vi "Teleop.vi"(10 "Match Info":T3={"Autonomous Elapsed Seconds"=0.0, "TeleOp Elapsed Seconds"=0.0, "Disabled Elapsed Seconds"=0.0, "Visited Autonomous"=FALSE, "Visited TeleOp"=FALSE, "Visited Disabled"=FALSE, "Autonomous Settings"={"Autonomous Style"=enum."Independent", "VI Refnum"=refnum}}, 11 "Call Context":T4) -> ()   [LabVIEW 2016]
doc: "This VI is called for each TeleOp packet received from the DS where the robot is not disabled. It is often used to read from the joysticks and update I/O or to update setpoints for timed control loops. It should complete and return within 20 milliseconds or it may miss DS packets."
uses:
  <vilib>/Rock Robotics/WPI/DriverStation/WPI_DriverStationDerivedRobotMode.ctl
  <vilib>/Rock Robotics/WPI/DriverStation/WPI_DriverStationMatch Info.ctl
  <vilib>/Rock Robotics/WPI/ThirdParty/Sensors/navX/_TypeDefs/FRIC_navX_DeviceNumbersTypeDef.ctl
  <vilib>/Rock Robotics/WPI/Solenoid/WPI_SolenoidValue.ctl
  <vilib>/Rock Robotics/WPI/Relay/WPI_RelayValue.ctl
  <vilib>/Rock Robotics/WPI/Utilities/WPI_GetSetVariantRefNum.vi
  <vilib>/Rock Robotics/WPI/Solenoid/WPI_SolenoidSetEnum.vi
  <vilib>/Rock Robotics/Network Tables/NT Write Boolean.vi
  <vilib>/Rock Robotics/Network Tables/NT Read Number.vi
  <vilib>/Rock Robotics/Network Tables/NT Write Number.vi
  Robot Global Data.vi
  driveCode/driveCodeTank.vi
  driveCode/driveCodeArcade.vi
  <vilib>/addons/control/pid/pid.llb/PID (DBL).vi
  <vilib>/addons/control/pid/NI_PID_pid.lvlib
panel:
  out "Yaw":dbl
  in  "graphs":enum32{"Shooter", "Drive", "Aiming"}(tab)
  out "shooterSpeed":dbl(graph)
  out "shooterVel":dbl
  out "driveChart":T1(graph)
  out "yaw":cluster{"Yaw":dbl, "angleToGoal":dbl}(graph)
  out "angleError":dbl
  in  "PID gains 2":T2={"proportional gain (Kc)"=0.008, "integral time (Ti, min)"=0.008, "derivative time (Td, min)"=0.0}
  in  "PID gains":T2={"proportional gain (Kc)"=0.009, "integral time (Ti, min)"=0.0, "derivative time (Td, min)"=0.011}
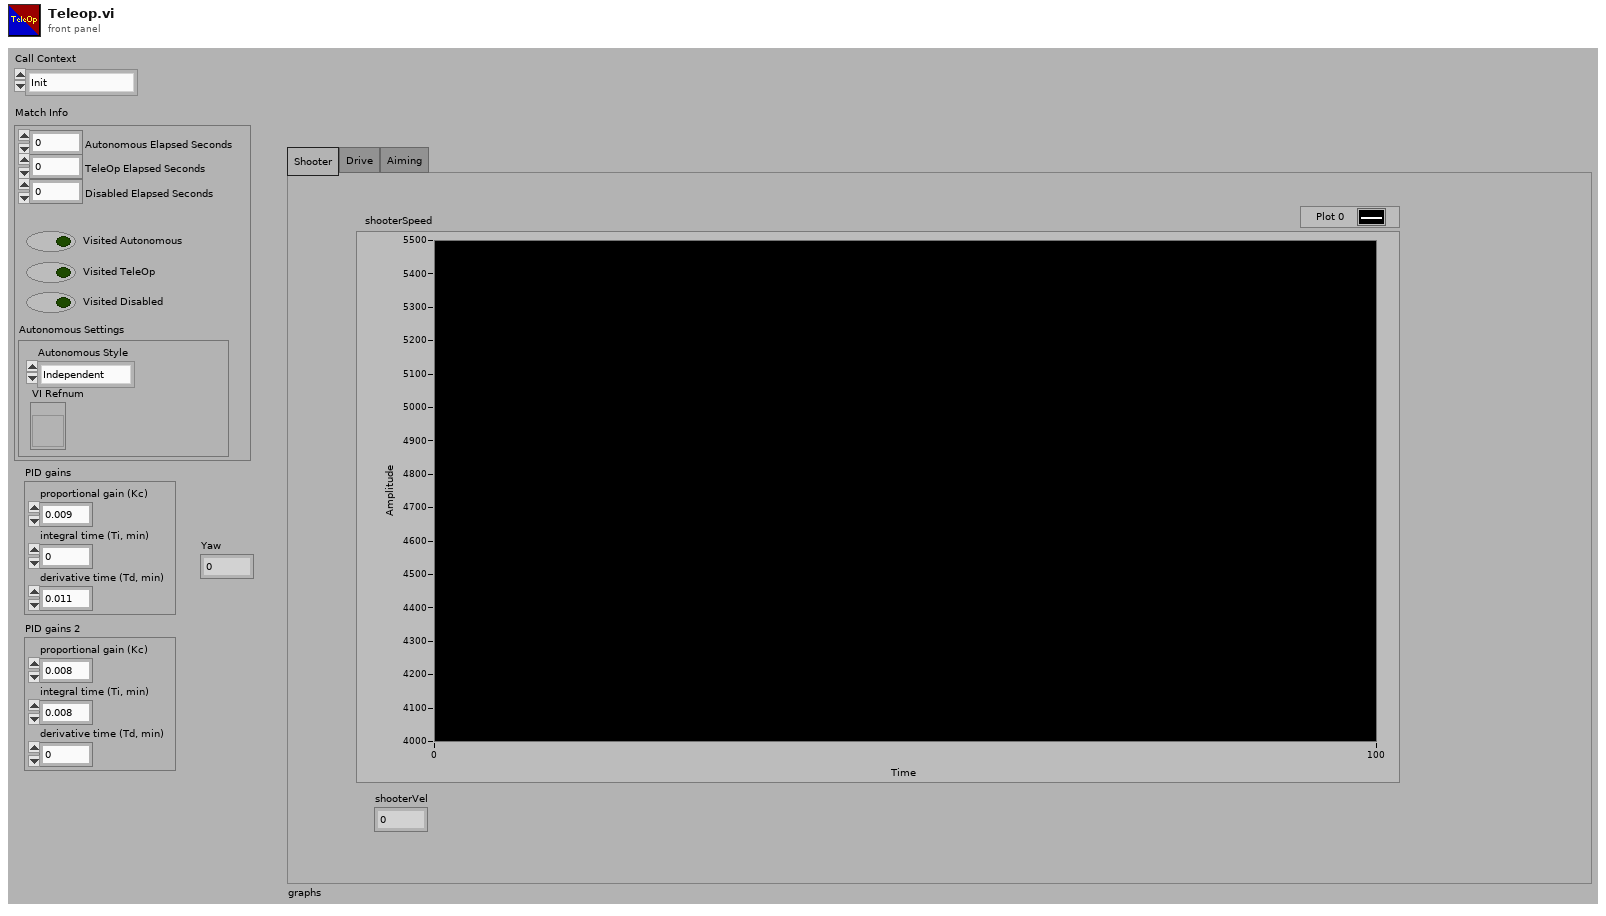
[diagram p1: front panel]
types:
  T1 = cluster{"Sensor Velocity":dbl, "Sensor Velocity":dbl}
  T2 = cluster{"proportional gain (Kc)":dbl, "integral time (Ti, min)":dbl, "derivative time (Td, min)":dbl}
  T3 = typedef "WPI_DriverStationMatch Info.ctl" = cluster{"Autonomous Elapsed Seconds":dbl, "TeleOp Elapsed Seconds":dbl, "Disabled Elapsed Seconds":dbl, "Visited Autonomous":bool, "Visited TeleOp":bool, "Visited Disabled":bool, "Autonomous Settings":cluster{"Autonomous Style":enum16{"Iterative", "Independent"}, "VI Refnum":refnum<vi>}}
  T4 = typedef "WPI_DriverStationDerivedRobotMode.ctl" = enum16{"Init", "Execute", "Stop"}
  T5 = typedef "WPI_SolenoidValue.ctl" = enum16{"Off", "On", "Forward", "Reverse"}
  T6 = typedef "FRIC_navX_DeviceNumbersTypeDef.ctl" = enum16{"Dev0", "Dev1", "Dev2", "Dev3"}
  T7 = typedef "WPI_JoystickDevRef.ctl" = cluster{"Device":T8}
  T8 = typedef "WPI_JoystickDeviceEnum.ctl" = enum16{"USB 0", "USB 1", "USB 2", "USB 3", "USB 4", "USB 5"}
  T9 = cluster{"Yaw":dbl, "Roll":dbl, "Pitch":dbl, "Heading":dbl, "Fused Heading":dbl}
  T10 = typedef "WPI_MotorControlDeviceRef.ctl" = cluster{"DeviceStatus":errorcluster, "Type":T11, "PWM":cluster{"PWM Channel":T12, "DeadBand":T13}, "CAN":cluster{"Device Number":u8, "SetOutput VI Ref":variant, "GetOutput VI Ref":variant, "Enable VI Ref":variant, "Disable VI Ref":variant, "Data":variant}, "Invert":bool}
  T11 = typedef "WPI_MotorControlType.ctl" = enum16{"PWM", "CAN"}
  T12 = typedef "FPGA_DIOPWMChannel.ctl" = enum8{"PWM 0", "PWM 1", "PWM 2", "PWM 3", "PWM 4", "PWM 5", "PWM 6", "PWM 7", "PWM 8", "PWM 9", "PWM MXP 0", "PWM MXP 1", "PWM MXP 2", "PWM MXP 3", "PWM MXP 4", "PWM MXP 5", "PWM MXP 6", "PWM MXP 7", "PWM MXP 8", "PWM MXP 9", "Invalid"}
  T13 = typedef "WPI_PWMDeadband.ctl" = cluster{"Name":string, "maxPositivePwm":i32, "minPositivePwm":i32, "centerPwm":i32, "maxNegativePwm":i32, "minNegativePwm":i32, "angularRange":u16}
  T14 = typedef "WPI_CANTalonSRX_GlobalStatus.ctl" = cluster{"Applied Throttle":dbl, "Module Enabled":bool, "CAN Error":errorcluster, "Closed Loop Error":dbl, "Forward Limit Switch Closed":bool, "Reverse Limit Switch Closed":bool, "Sensor Position":dbl, "Sensor Velocity":dbl, "Current":dbl, "Sticky Fault - Over Temp":bool, "Sticky Fault - Under Voltage":bool, "Sticky Fault - Forward Limit":bool, "Sticky Fault - Reverse Limit":bool, "Sticky Fault - Forward Soft Limit":bool, "Sticky Fault - Reverse Soft Limit":bool, "Brake is Enabled":bool, "Encoder Position":dbl, "Encoder Velocity":dbl, "Encoder Index Count":dbl, "Encoder A Pin State":bool, "Encoder B Pin State":bool, "Encoder Index Pin State":bool, "Analog In":dbl, "Analog In Velocity":dbl, "Temperature (C)":dbl, "Battery Voltage":dbl, "Control 5 Is Supported":bool, "Current Profile Slot Select":dbl, "Pos Div 8":bool, "Vel Div 4":bool, "Pulse Width Position":i32, "Pulse Width Velocity":i32, "Pulse Width Rise To Rise (us)":i32, "Pulse Width Rise To Fall (us)":i32, "Mot Prof Active Is Under Run":bool, "Mot Prof Active Has Under Run":bool, "Mot Prof Active Is Last":bool, "Mot Prof Active Velocity Only":bool, "Mot Prof Active Is Valid":bool, "Mot Prof Buffer Is Full":bool, "Mot Prof Active Profile Slot Select":i32, "Mot Prof NextID":i32, "Mot Prof Count":i32, "Mot Prof Active Velocity":dbl, "Mot Prof Active Position":dbl, "Mot Prof Output Enable":i32}
  T15 = typedef "WPI_CompressorDevRef.ctl" = cluster{"DevStatus":errorcluster, "Pneumatics Control Module":u8}
  T16 = typedef "WPI_RelayDevRef.ctl" = cluster{"DevStatus":errorcluster, "Relay Channel":T17, "Relay Direction":T18}
  T17 = typedef "FPGA_DIORelayChannel.ctl" = enum8{"Relay 0", "Relay 1", "Relay 2", "Relay 3", "Invalid"}
  T18 = typedef "WPI_RelayDirection.ctl" = enum16{"Both directions", "Forward only", "Reverse only"}
  T19 = typedef "WPI_RelayValue.ctl" = enum16{"Off", "On", "Forward", "Reverse"}
  T20 = typedef "WPI_SolenoidDevRef.ctl" = cluster{"DevStatus":errorcluster, "Pneumatics Control Module":u8, "Forward Solenoid Channel":T21, "Reverse Solenoid Channel":T21}
  T21 = typedef "WPI_SolenoidChannel.ctl" = enum8{"Solenoid 0", "Solenoid 1", "Solenoid 2", "Solenoid 3", "Solenoid 4", "Solenoid 5", "Solenoid 6", "Solenoid 7", "Invalid"}
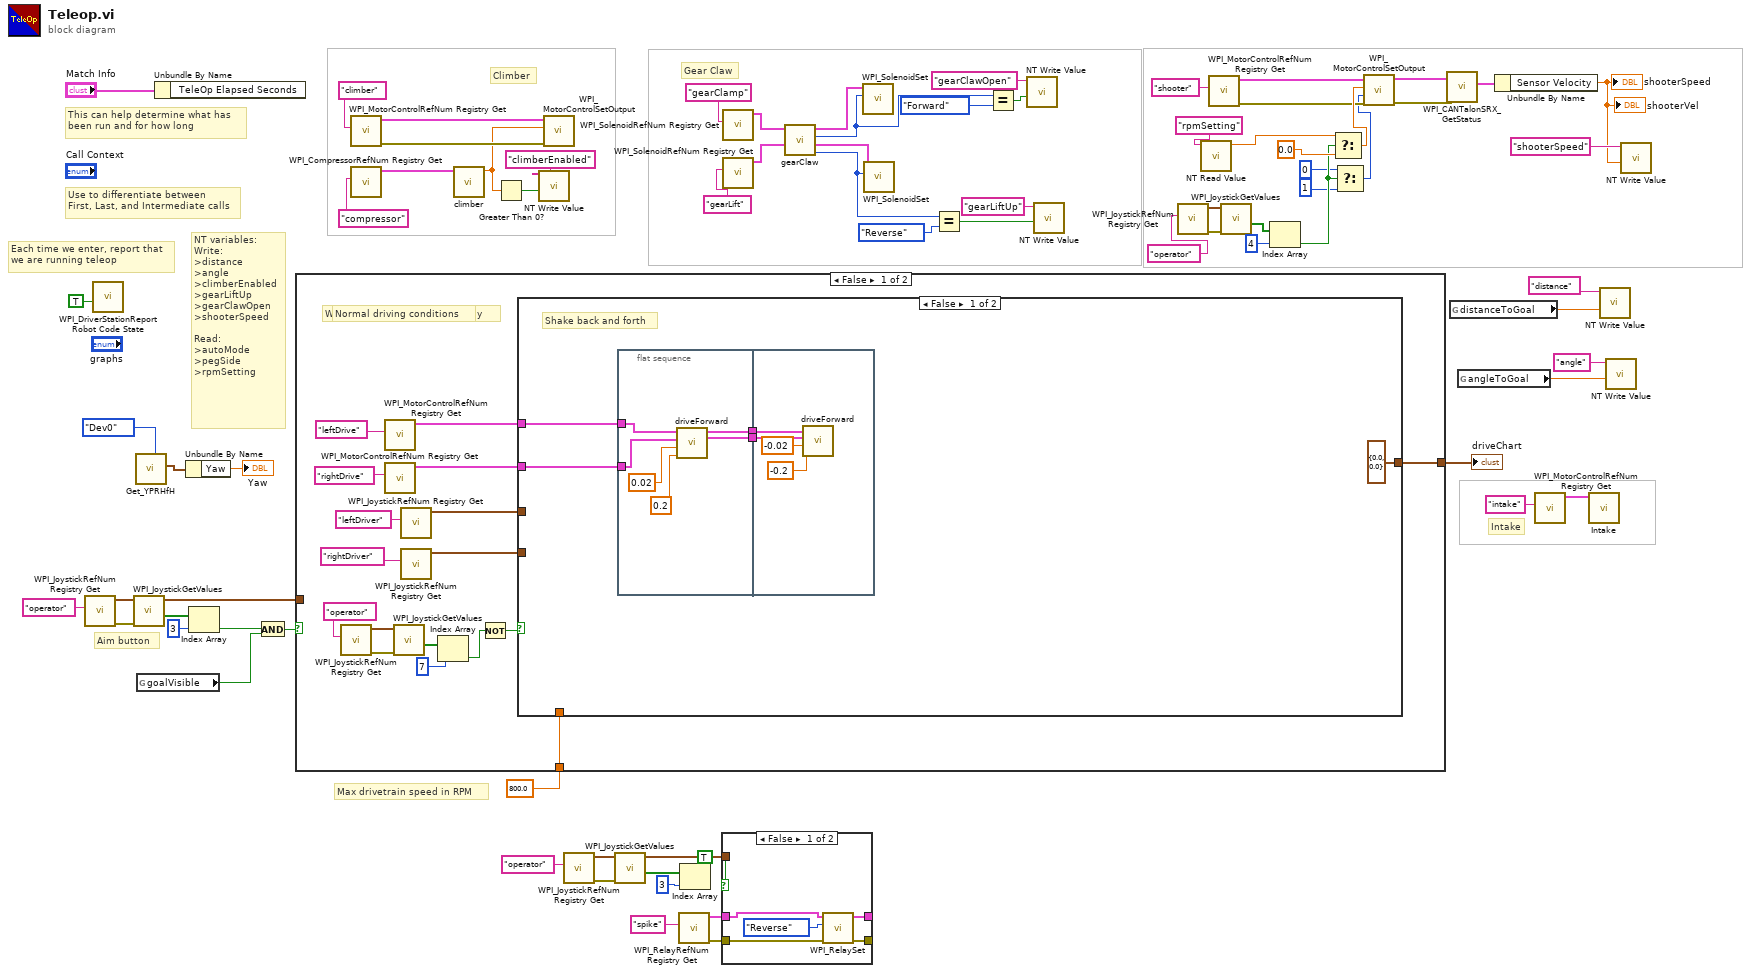
[diagram p0: block diagram]
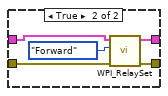
[diagram p2: hidden frame]
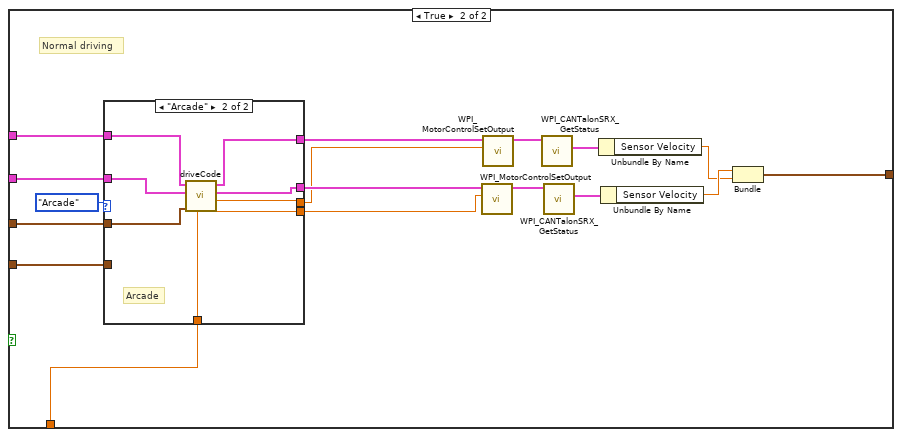
[diagram p3: hidden frame]
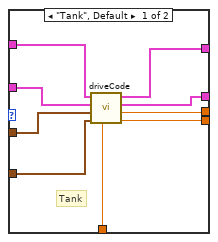
[diagram p4: hidden frame]
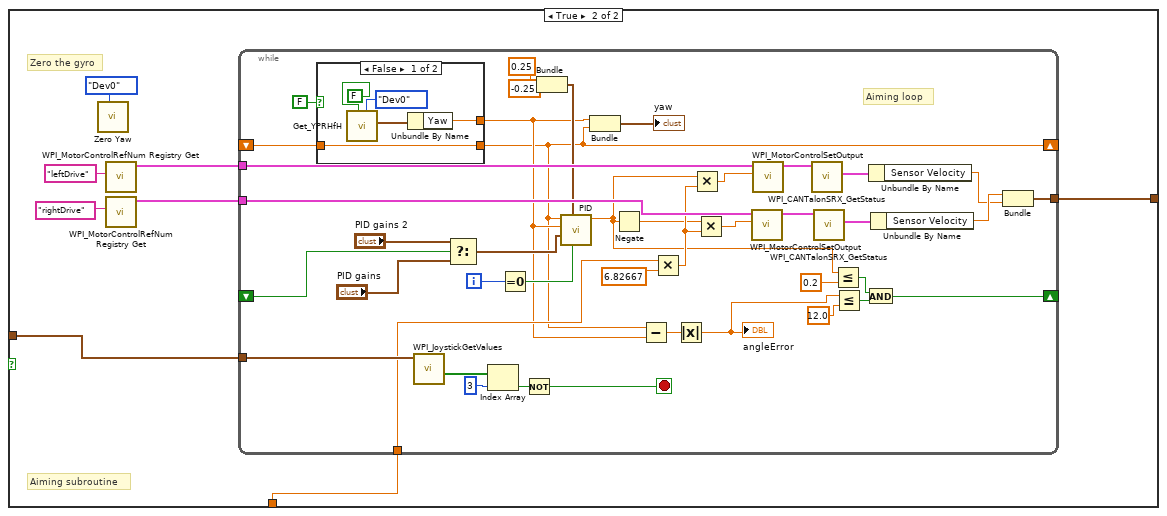
[diagram p5: hidden frame]
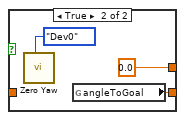
[diagram p6: hidden frame]
diagram:
  # "NT variables:\nWrite:\n>distance\n>angle\n>climberEnabled\n>gearLiftUp\n>gearClawOpen\n>shooterSpeed\n\nRead:\n>autoMode\n>pegSide\n>rpmSetting"
  # "Gear Claw"
  # "Max drivetrain speed in RPM"
  # "Aim button"
  # "Intake"
  # "Climber"
  # "Each time we enter, report that\nwe are running teleop"
  # "Use to differentiate between\nFirst, Last, and Intermediate calls"
  # "This can help determine what has\nbeen run and for how long"
  n1 = call <vilib>:"WPI_JoystickRefNum Registry Get.vi"("refnum name"="operator") -> ("error out"=w63:errorcluster, "JoystickDevRef"=w62:T7)  [unwired: 9 in]
  n2 = call <vilib>:"WPI_DriverStationReport Robot Code State.vi"("TeleOp"=TRUE ("Autonomous")) -> ()  [unwired: 10 in, 1 out]
  n3 = call <vilib>:"WPI_JoystickGetValues.vi"("error in (no error)"=w63, "JoystickDevRef"=w62) -> ("Buttons"=w61:bool[], "JoystickDevRef"=w58:T7)  [unwired: 5 in, 3 out]
  n4 = call <vilib>:"Get_YPRHfH.vi"("Device Number"=FRIC_navX_DeviceNumbersTypeDef."Dev0") -> ("YRPHfH"=w39:T9)  [unwired: 10 in]
  n5 = global read "Robot Global Data.vi" "goalVisible"() -> (w55:bool)
  n6 = Unbundle By Name("Match Info") -> ()  [unwired: 1 out]
  n7 = Unbundle By Name(w39) -> ("Yaw"=→"Yaw":dbl)
  n8 = Index Array(array=w61, index=3) -> (element=w56:bool)
  n9 = And(x=w56, y=w55) -> (x .and. y?=w57:bool)
  n10 = case shown="False" w57 {
    tunnel: [w85 w149] -> w70
    tunnel: 800.0 ("maxSpeed") -> [w83 w147]
    tunnel: w58 -> [_ w148]
    frame False {
      # "When not aiming, drive normally"
      # "Normal driving conditions"
      n11 = call <vilib>:"WPI_JoystickRefNum Registry Get.vi"("refnum name"="operator") -> ("error out"=w80:errorcluster, "JoystickDevRef"=w81:T7)  [unwired: 9 in]
      n12 = call <vilib>:"WPI_MotorControlRefNum Registry Get.vi"("refnum name"="leftDrive") -> ("MotorControlDevRef"=w86:T10)  [unwired: 9 in, 1 out]
      n13 = call <vilib>:"WPI_MotorControlRefNum Registry Get.vi"("refnum name"="rightDrive") -> ("MotorControlDevRef"=w84:T10)  [unwired: 9 in, 1 out]
      n14 = call <vilib>:"WPI_JoystickGetValues.vi"("error in (no error)"=w80, "JoystickDevRef"=w81) -> ("Buttons"=w79:bool[])  [unwired: 5 in, 4 out]
      n15 = call <vilib>:"WPI_JoystickRefNum Registry Get.vi"("refnum name"="leftDriver") -> ("JoystickDevRef"=w88:T7)  [unwired: 9 in, 1 out]
      n16 = call <vilib>:"WPI_JoystickRefNum Registry Get.vi"("refnum name"="rightDriver") -> ("JoystickDevRef"=w87:T7)  [unwired: 9 in, 1 out]
      n17 = Index Array(array=w79, index=7) -> (element=w76:bool)
      n18 = Not(x=w76) -> (.not. x?=w77:bool)
      n19 = case shown="False" w77 {
        tunnel: w88 -> [_ w124]
        tunnel: w87 -> [_ w123]
        tunnel: w86 -> [w97 w119]
        tunnel: [T1 {"Sensor Velocity"=0.0, "Sensor Velocity"=0.0} w115] -> w85
        tunnel: w84 -> [w96 w112]
        tunnel: w83 -> [_ w111]
        frame False {
          # "Shake back and forth"
          n20 = flat-sequence {
            tunnel: w97 -> [w103]
            tunnel: w96 -> [w102]
            tunnel: [w99] -> w95
            tunnel: [w98] -> w94
            tunnel: w95 -> [w107]
            tunnel: w94 -> [w106]
            frame #0 {
              n21 = call "driveForward.vi"("speed (%)"=0.2, "distance (ft)"=0.02, "rightMotor"=w102, "leftMotor"=w103) -> ("rightMotor"=w98:T10, "leftMotor"=w99:T10)  [unwired: 6 in]
            }
            frame #1 {
              n22 = call "driveForward.vi"("speed (%)"=-0.2, "distance (ft)"=-0.02, "rightMotor"=w106, "leftMotor"=w107) -> ()  [unwired: 6 in, 2 out]
            }
          }
        }
        frame True {
          # "Normal driving"
          n23 = case shown="\"Arcade\"" enum16{"Arcade", "Tank"}."Arcade" {
            tunnel: w119 -> [w133 w141]
            tunnel: w124 -> [w132 w136]
            tunnel: w123 -> [w125 _]
            tunnel: [w131 w140] -> w122
            tunnel: [w130 w139] -> w121
            tunnel: [w129 w138] -> w110
            tunnel: [w128 w137] -> w109
            tunnel: w112 -> [w127 w134]
            tunnel: w111 -> [w126 w135]
            frame "Tank", Default {
              # "Tank"
              n24 = call-poly "driveCode.vi"("maxSpeed"=w126, "rightJoystick"=w125, "leftJoystick"=w132, "rightDrive"=w127, "leftDrive"=w133) -> ("rightSpeed"=w128:dbl, "leftSpeed"=w129:dbl, "rightDrive"=w130:T10, "leftDrive"=w131:T10)  [unwired: 3 in]
            }
            frame "Arcade" {
              # "Arcade"
              n25 = call-poly "driveCode.vi"("maxSpeed"=w135, "joystick"=w136, "rightMotor"=w134, "leftMotor"=w141) -> ("rightSpeed"=w137:dbl, "leftSpeed"=w138:dbl, "rightMotor"=w139:T10, "leftMotor"=w140:T10)  [unwired: 4 in]
            }
          }
          n26 = call <vilib>:"WPI_MotorControlSetOutput.vi"("Output"=w109, "MotorControlDevRef"=w121) -> ("MotorControlDevRef"=w118:T10)  [unwired: 7 in, 2 out]
          n27 = call <vilib>:"WPI_MotorControlSetOutput.vi"("Output"=w110, "MotorControlDevRef"=w122) -> ("MotorControlDevRef"=w116:T10)  [unwired: 7 in, 2 out]
          n28 = call <vilib>:"WPI_CANTalonSRX_GetStatus.vi"("CAN Talon SRX Ref"=w116) -> ("Talon SRX Status"=w117:T14)  [unwired: 8 in, 2 out]
          n29 = call <vilib>:"WPI_CANTalonSRX_GetStatus.vi"("CAN Talon SRX Ref"=w118) -> ("Talon SRX Status"=w120:T14)  [unwired: 8 in, 2 out]
          n30 = Unbundle By Name(w117) -> ("Sensor Velocity"=w113:dbl)
          n31 = Unbundle By Name(w120) -> ("Sensor Velocity"=w114:dbl)
          n32 = Bundle("Sensor Velocity"=w114, "Sensor Velocity"=w113) -> (w115:T1)  [unwired: 1 in]
        }
      }
    }
    frame True {
      # "Zero the gyro"
      # "Aiming subroutine"
      n33 = call <vilib>:"Zero Yaw.vi"("Device Number"=FRIC_navX_DeviceNumbersTypeDef."Dev0") -> ()  [unwired: 11 in]
      n34 = call <vilib>:"WPI_MotorControlRefNum Registry Get.vi"("refnum name"="leftDrive") -> ("MotorControlDevRef"=w144:T10)  [unwired: 9 in, 1 out]
      n35 = call <vilib>:"WPI_MotorControlRefNum Registry Get.vi"("refnum name"="rightDrive") -> ("MotorControlDevRef"=w143:T10)  [unwired: 9 in, 1 out]
      n36 = while {
        tunnel: [w191] -> w149
        tunnel: w144 -> [w190]
        tunnel: w143 -> [w189]
        tunnel: w148 -> [w188]
        tunnel: w147 -> [w187]
        shift-right: [w184] -> _
        shift-left: _ -> [w183]
        shift-right: [w152] -> _
        shift-left: _ -> [w154]
        i -> [w186]
        stop <- w185 stop-if-true
        # "Aiming loop"
        n37 = case shown="False" FALSE {
          tunnel: [w193 0.0] -> w157
          tunnel: [w192 w197] -> w152
          tunnel: w154 -> [w192 _]
          frame False {
            n38 = call <vilib>:"Get_YPRHfH.vi"("Device Number"=FRIC_navX_DeviceNumbersTypeDef."Dev0", "Update"=FALSE) -> ("YRPHfH"=w196:T9)  [unwired: 9 in]
            n39 = Unbundle By Name(w196) -> ("Yaw"=w193:dbl)
          }
          frame True {
            n40 = call <vilib>:"Zero Yaw.vi"("Device Number"=FRIC_navX_DeviceNumbersTypeDef."Dev0") -> ()  [unwired: 11 in]
            n41 = global read "Robot Global Data.vi" "angleToGoal"() -> (w197:dbl)
          }
        }
        n42 = call <vilib>:"WPI_JoystickGetValues.vi"("JoystickDevRef"=w188) -> ("Buttons"=w175:bool[])  [unwired: 6 in, 4 out]
        n43 = Select(t="PID gains 2", s=w183, f="PID gains") -> (s? t:f=w162:T2)
        n44 = Index Array(array=w175, index=3) -> (element=w174:bool)
        n45 = Equal To 0?(x=w186) -> (x = 0?=w161:bool)
        n46 = Not(x=w174) -> (.not. x?=w185:bool)
        n47 = Bundle(0.25, -0.25) -> (w160:cluster{dbl, dbl})  [unwired: 1 in]
        n48 = call-poly <vilib>:"PID.vi"("reinitialize? (F)"=w161, "output range"=w160, "PID gains"=w162, "process variable"=w157, "setpoint"=w152) -> ("output"=w151:dbl)  [unwired: 5 in, 1 out]
        n49 = Bundle("Yaw"=w157, "angleToGoal"=w152) -> (→"yaw":cluster{"Yaw":dbl, "angleToGoal":dbl})  [unwired: 1 in]
        n50 = Negate(x=w151) -> (-x=w159:dbl)
        n51 = Subtract(x=w152, y=w157) -> (x-y=w158:dbl)
        n52 = Multiply(x=w187, y=6.82667) -> (x*y=w172:dbl)
        n53 = Absolute Value(x=w158) -> (abs(x)=w156:dbl)
        "angleError" <- w156
        n54 = Multiply(x=w151, y=w172) -> (x*y=w155:dbl)
        n55 = Multiply(x=w159, y=w172) -> (x*y=w173:dbl)
        n56 = call <vilib>:"WPI_MotorControlSetOutput.vi"("Output"=w173, "MotorControlDevRef"=w189) -> ("MotorControlDevRef"=w181:T10)  [unwired: 7 in, 2 out]
        n57 = call <vilib>:"WPI_MotorControlSetOutput.vi"("Output"=w155, "MotorControlDevRef"=w190) -> ("MotorControlDevRef"=w179:T10)  [unwired: 7 in, 2 out]
        n58 = call <vilib>:"WPI_CANTalonSRX_GetStatus.vi"("CAN Talon SRX Ref"=w179) -> ("Talon SRX Status"=w180:T14)  [unwired: 8 in, 2 out]
        n59 = call <vilib>:"WPI_CANTalonSRX_GetStatus.vi"("CAN Talon SRX Ref"=w181) -> ("Talon SRX Status"=w182:T14)  [unwired: 8 in, 2 out]
        n60 = Less Or Equal?(x=w151, y=0.2) -> (x <= y?=w166:bool)
        n61 = Less Or Equal?(x=w156, y=12.0) -> (x <= y?=w167:bool)
        n62 = And(x=w166, y=w167) -> (x .and. y?=w184:bool)
        n63 = Unbundle By Name(w180) -> ("Sensor Velocity"=w177:dbl)
        n64 = Unbundle By Name(w182) -> ("Sensor Velocity"=w178:dbl)
        n65 = Bundle("Sensor Velocity"=w178, "Sensor Velocity"=w177) -> (w191:T1)  [unwired: 1 in]
      }
    }
  }
  "driveChart" <- w70
  n66 = call <vilib>:"WPI_MotorControlRefNum Registry Get.vi"("refnum name"="climber") -> ("error out"=w72:errorcluster, "MotorControlDevRef"=w73:T10)  [unwired: 9 in]
  n67 = call <vilib>:"WPI_CompressorRefNum Registry Get.vi"("refnum name"="compressor") -> ("CompressorDevRef"=w68:T15)  [unwired: 9 in, 1 out]
  n68 = call "climber.vi"("compressorDev"=w68) -> ("motorSpeed"=w31:dbl)  [unwired: 10 in]
  n69 = Greater Than 0?(x=w31) -> (x > 0?=w30:bool)
  n70 = call-poly <vilib>:"NT Write Value.vi"("Boolean"=w30, "Name"="climberEnabled") -> ()  [unwired: 9 in, 1 out]
  n71 = call <vilib>:"WPI_MotorControlSetOutput.vi"("error in (no error)"=w72, "Output"=w31, "MotorControlDevRef"=w73) -> ()  [unwired: 6 in, 3 out]
  n72 = call <vilib>:"WPI_JoystickRefNum Registry Get.vi"("refnum name"="operator") -> ("error out"=w3:errorcluster, "JoystickDevRef"=w4:T7)  [unwired: 9 in]
  n73 = call <vilib>:"WPI_JoystickGetValues.vi"("error in (no error)"=w3, "JoystickDevRef"=w4) -> ("Buttons"=w10:bool[], "JoystickDevRef"=w5:T7)  [unwired: 5 in, 3 out]
  n74 = call <vilib>:"WPI_RelayRefNum Registry Get.vi"("refnum name"="spike") -> ("error out"=w6:errorcluster, "RelayDevRef"=w7:T16)  [unwired: 9 in]
  n75 = Index Array(array=w10, index=3) -> ()  [unwired: 1 out]
  n76 = case shown="False" TRUE {
    tunnel: [w203 w208] -> _
    tunnel: [w202 w207] -> _
    tunnel: w7 -> [w201 w206]
    tunnel: w6 -> [w200 w205]
    tunnel: w5 -> [_ _]
    frame False {
      n77 = call <vilib>:"WPI_RelaySet.vi"("error in (no error)"=w200, "RelayValue"=WPI_RelayValue."Reverse", "RelayDevRef"=w201) -> ("error out"=w202:errorcluster, "RelayDevRef"=w203:T16)  [unwired: 7 in]
    }
    frame True {
      n78 = call <vilib>:"WPI_RelaySet.vi"("error in (no error)"=w205, "RelayValue"=WPI_RelayValue."Forward", "RelayDevRef"=w206) -> ("error out"=w207:errorcluster, "RelayDevRef"=w208:T16)  [unwired: 7 in]
    }
  }
  n79 = call <vilib>:"WPI_SolenoidRefNum Registry Get.vi"("refnum name"="gearClamp") -> ("SolenoidDevRef"=w52:T20)  [unwired: 9 in, 1 out]
  n80 = call <vilib>:"WPI_SolenoidRefNum Registry Get.vi"("refnum name"="gearLift") -> ("SolenoidDevRef"=w51:T20)  [unwired: 9 in, 1 out]
  n81 = call "gearClaw.vi"("lifter"=w51, "clamper"=w52) -> ("lifterValue"=w24:T5, "lifter"=w50:T20, "clamperValue"=w19:T5, "clamper"=w49:T20)  [unwired: 6 in]
  n82 = call-poly <vilib>:"WPI_SolenoidSet.vi"("Value"=w19, "SolenoidDevRef"=w49) -> ()  [unwired: 8 in, 2 out]
  n83 = call-poly <vilib>:"WPI_SolenoidSet.vi"("Value"=w24, "SolenoidDevRef"=w50) -> ()  [unwired: 8 in, 2 out]
  n84 = Equal?(x=w24, y=WPI_SolenoidValue."Reverse" ("lifterValue")) -> (x = y?=w25:bool)
  n85 = Equal?(x=w19, y=WPI_SolenoidValue."Forward" ("lifterValue")) -> (x = y?=w20:bool)
  n86 = call-poly <vilib>:"NT Write Value.vi"("Boolean"=w20, "Name"="gearClawOpen") -> ()  [unwired: 9 in, 1 out]
  n87 = call-poly <vilib>:"NT Write Value.vi"("Boolean"=w25, "Name"="gearLiftUp") -> ()  [unwired: 9 in, 1 out]
  n88 = call <vilib>:"WPI_JoystickRefNum Registry Get.vi"("refnum name"="operator") -> ("error out"=w45:errorcluster, "JoystickDevRef"=w44:T7)  [unwired: 9 in]
  n89 = call-poly <vilib>:"NT Read Value.vi"("Name"="rpmSetting") -> ("Numeric"=w17:dbl)  [unwired: 9 in, 1 out]
  n90 = call <vilib>:"WPI_MotorControlRefNum Registry Get.vi"("refnum name"="shooter") -> ("error out"=w15:errorcluster, "MotorControlDevRef"=w16:T10)  [unwired: 9 in]
  n91 = call <vilib>:"WPI_JoystickGetValues.vi"("error in (no error)"=w45, "JoystickDevRef"=w44) -> ("Buttons"=w43:bool[])  [unwired: 5 in, 4 out]
  n92 = Index Array(array=w43, index=4) -> (element=w14:bool)
  n93 = Select(t=w17, s=w14, f=0.0) -> (s? t:f=w41:dbl)
  n94 = Select(t=u8 0 ("options"), s=w14, f=u8 1 ("options")) -> (s? t:f=w13:u8)
  n95 = call <vilib>:"WPI_MotorControlSetOutput.vi"("error in (no error)"=w15, "options"=w13, "Output"=w41, "MotorControlDevRef"=w16) -> ("error out"=w47:errorcluster, "MotorControlDevRef"=w48:T10)  [unwired: 5 in, 1 out]
  n96 = call <vilib>:"WPI_CANTalonSRX_GetStatus.vi"("error in (no error)"=w47, "CAN Talon SRX Ref"=w48) -> ("Talon SRX Status"=w36:T14)  [unwired: 7 in, 2 out]
  n97 = global read "Robot Global Data.vi" "distanceToGoal"() -> (w32:dbl)
  n98 = global read "Robot Global Data.vi" "angleToGoal"() -> (w33:dbl)
  n99 = Unbundle By Name(w36) -> ("Sensor Velocity"=w18:dbl)
  "shooterVel" <- w18
  "shooterSpeed" <- w18
  n100 = call <vilib>:"WPI_MotorControlRefNum Registry Get.vi"("refnum name"="intake") -> ("MotorControlDevRef"=w67:T10)  [unwired: 9 in, 1 out]
  n101 = call "Intake.vi"("intake"=w67) -> ()  [unwired: 11 in]
  n102 = call-poly <vilib>:"NT Write Value.vi"("Numeric"=w32, "Name"="distance") -> ()  [unwired: 9 in, 1 out]
  n103 = call-poly <vilib>:"NT Write Value.vi"("Numeric"=w33, "Name"="angle") -> ()  [unwired: 9 in, 1 out]
  n104 = call-poly <vilib>:"NT Write Value.vi"("Numeric"=w18, "Name"="shooterSpeed") -> ()  [unwired: 9 in, 1 out]
